vi "3DStyle.vi"(10 "Style":T2) -> (2 "Scatter Point Style":T1)   [LabVIEW 2020]
uses:
  _Controls/Style.ctl
  <vilib>/Math Plots/3D Math Plots/3D Plot/3D Plot/Typedef/Sprite Type.ctl
  <vilib>/Math Plots/3D Math Plots/3D Plot/3D Plot/3D Plot.lvclass
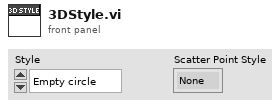
[diagram p1: front panel]
types:
  T1 = typedef "3D Plot.lvclass/Sprite Type.ctl" = enum16{"None", "Empty Square", "Solid Square", "Empty Diamond", "Solid Diamond", "Empty Circle", "Solid Circle", "Asterisk", "Bold X", "Wireframe Sphere", "Solid Sphere", "Wireframe Cube", "Solid Cube"}
  T2 = typedef "Style.ctl" = enum16{"Empty circle", "Full circle", "Empty square", "Full square", "Cross"}
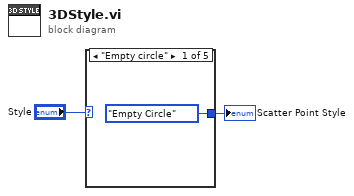
[diagram p0: block diagram]
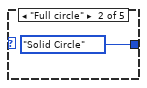
[diagram p2: hidden frame]
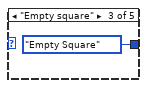
[diagram p3: hidden frame]
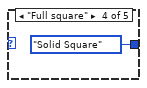
[diagram p4: hidden frame]
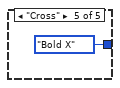
[diagram p5: hidden frame]
diagram:
  n1 = case shown="\"Empty circle\"" "Style" {
    tunnel: [Sprite_Type."Empty Circle" ("Plot Specific:Scatter:Scatter Point Style") Sprite_Type."Solid Circle" ("Plot Specific:Scatter:Scatter Point Style") Sprite_Type."Empty Square" ("Plot Specific:Scatter:Scatter Point Style") Sprite_Type."Solid Square" ("Plot Specific:Scatter:Scatter Point Style") Sprite_Type."Bold X" ("Plot Specific:Scatter:Scatter Point Style")] -> w1
    frame "Empty circle" {
    }
    frame "Full circle" {
    }
    frame "Empty square" {
    }
    frame "Full square" {
    }
    frame "Cross" {
    }
  }
  "Scatter Point Style" <- w1
